vi "Get Category.vi"(8 "error in (no error)":errorcluster, 11 "UI Reference editor node in":refnum<class "UI Reference editor node.lvclass">) -> (0 "error out":errorcluster, 2 "Category":string, 3 "UI Reference editor node out":refnum<class "UI Reference editor node.lvclass">)   [LabVIEW 2015, in "UI Reference editor node.lvclass"]
uses:
  UI Reference editor node.lvclass
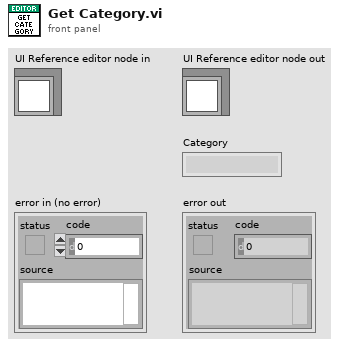
[diagram p1: front panel]
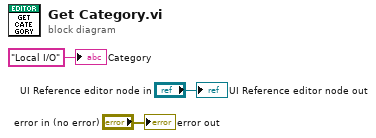
[diagram p0: block diagram]
diagram:
  "error out" <- "error in (no error)"
  "UI Reference editor node out" <- "UI Reference editor node in"
  "Category" <- "Local I/O" ("Category")
